vi "Express XY Graph.vi"() -> ()   [LabVIEW 2010]
uses:
  Instance           6 24Saved   Express XY Graph .vi
  Instance           2 24Saved   Express XY Graph .vi
  Instance           4 24Saved   Express XY Graph .vi
  Instance           5 24Saved   Express XY Graph .vi
  Instance           1 24Saved   Express XY Graph .vi
  Instance           3 24Saved   Express XY Graph .vi
  <vilib>/Analysis/NI_AALBase.lvlib
panel:
  out "XY图":cluster{"Y":dbl[], "Y":dbl[]}[](graph)
  out "XY图":cluster{"Y":dbl[], "Y":dbl[]}[](graph)
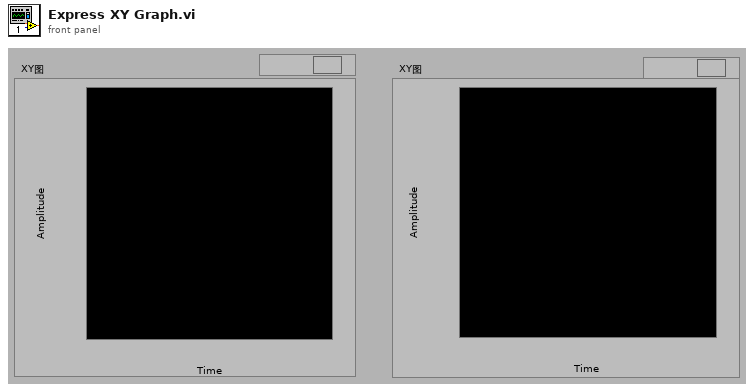
[diagram p1: front panel]
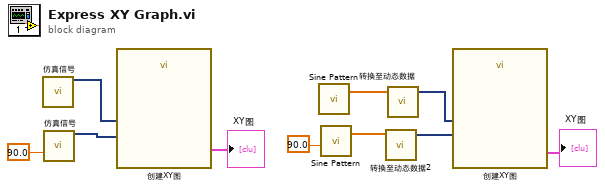
[diagram p0: block diagram]
diagram:
  n1 = call "仿真信号"() -> ("正弦"=w9:dynamicdata)  [unwired: 14 in, 1 out]
  n2 = call "仿真信号"("Phase"=90.0) -> ("正弦"=w8:dynamicdata)  [unwired: 13 in, 1 out]
  n3 = call "创建XY图"("Y Input"=w8, "X Input"=w9) -> ("XY Graph"=→"XY图":cluster{"Y":dbl[], "Y":dbl[]}[])  [unwired: 8 in, 1 out]
  n4 = call <vilib>:"Sine Pattern.vi"() -> ("Sinusoidal Pattern"=w6:dbl[])  [unwired: 4 in, 1 out]
  n5 = call <vilib>:"Sine Pattern.vi"("phase(degrees)"=90.0) -> ("Sinusoidal Pattern"=w5:dbl[])  [unwired: 3 in, 1 out]
  n6 = call "转换至动态数据2"("Array"=w5) -> ("Dynamic Data Type"=w3:dynamicdata)  [unwired: 3 in]
  n7 = call "转换至动态数据"("Array"=w6) -> ("Dynamic Data Type"=w4:dynamicdata)  [unwired: 3 in]
  n8 = call "创建XY图"("Y Input"=w3, "X Input"=w4) -> ("XY Graph"=→"XY图":cluster{"Y":dbl[], "Y":dbl[]}[])  [unwired: 8 in, 1 out]
